vi "Get Channel UIs.vi"(8 "error in (no error)":errorcluster, 11 "Component UI in":refnum<class "Component User Interfaces.lvclass">) -> (0 "error out":errorcluster, 1 "Tx Channel UI":refnum<class "User Interface.lvclass">, 2 "Rx Channel UI":refnum<class "User Interface.lvclass">, 3 "Component UI out":refnum<class "Component User Interfaces.lvclass">)   [LabVIEW 2017, in "DSF Core.lvlib" / "Component User Interfaces.lvclass"]
uses:
  Component User Interfaces.lvclass
  User Interface/User Interface.lvclass
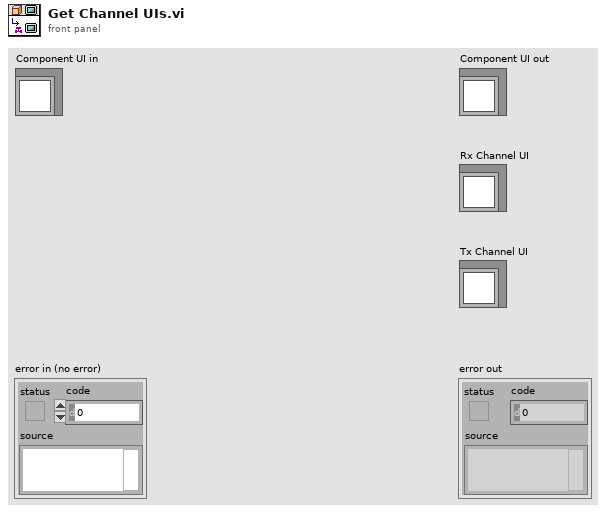
[diagram p1: front panel]
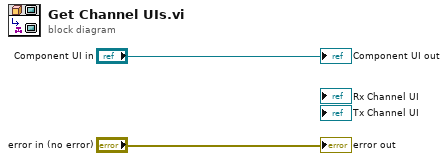
[diagram p0: block diagram]
diagram:
  "error out" <- "error in (no error)"
  "Component UI out" <- "Component UI in"
